vi "SLSC Add Status Section.vi"(5 "GUID Channel Interface":string="03D3BB89-1485-13A6-56005DE6430FF8B7", 6 "SLSC Channel Path":string="SLSCChannelPath", 7 "GUID (Default Section)":string="03D3BB89-1485-13A6-56005DE6430FF8B7", 8 "error in (no error)":errorcluster, 9 "Outgoing configuration":T3(array[cluster]), 10 "Section Name":string, 11 "Parent Ref in":T4 format="%.0x") -> (0 "error out":errorcluster, 3 "Parent Ref out":T4 format="%.0x")   [LabVIEW 2017, in "SLSC CD System Explorer.lvlib"]
uses:
  SLSC CD System Explorer.lvlib
  <vilib>/NI Veristand/Custom Device API/Custom Device Item Ref.ctl
  <vilib>/NI Veristand/Custom Device API/Custom Device Channel.ctl
  <vilib>/NI Veristand/Custom Device API/Custom Device Channel Type.ctl
  <vilib>/NI Veristand/Custom Device API/Set Item Property (String).vi
  <vilib>/NI VeriStand/Custom Device API/Custom Device API.lvlib
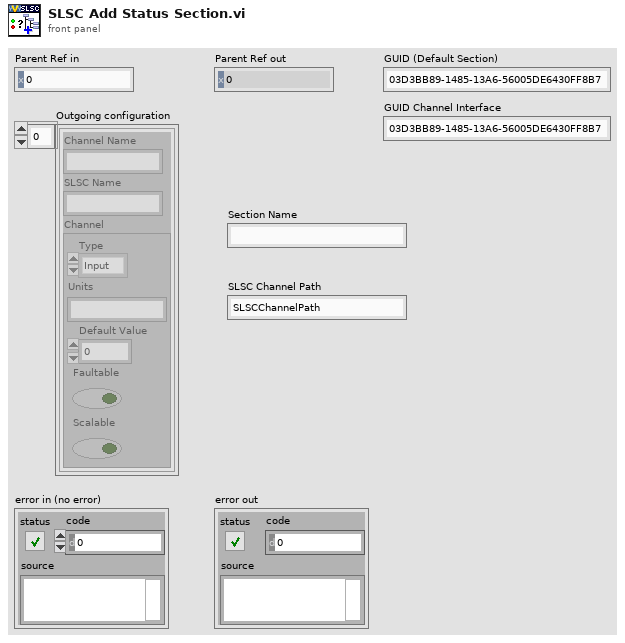
[diagram p1: front panel]
types:
  T1 = typedef "Custom Device API.lvlib/Custom Device Channel.ctl" = cluster{"Type":T2, "Units":string, "Default Value":dbl, "Faultable":bool, "Scalable":bool}
  T2 = typedef "Custom Device API.lvlib/Custom Device Channel Type.ctl" = enum16{"Input", "Output"}
  T3 = cluster{"Channel Name":string, "SLSC Name":string, "Channel":T1}[]
  T4 = typedef "Custom Device API.lvlib/Custom Device Item Ref.ctl" = u64
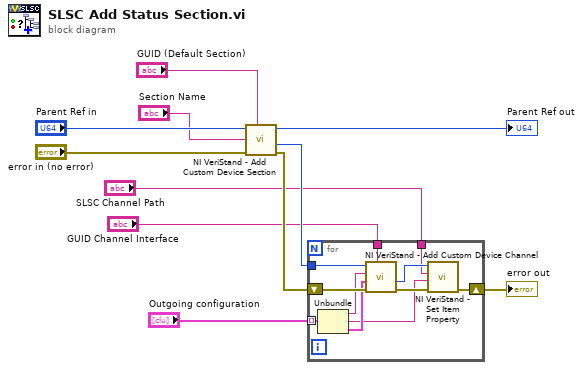
[diagram p0: block diagram]
diagram:
  n1 = call <vilib>:"NI VeriStand - Add Custom Device Section.vi"("GUID (Default Section)"="GUID (Default Section)", "error in (no error)"="error in (no error)", "Section Name"="Section Name", "Parent Ref in"="Parent Ref in") -> ("error out"=w5:errorcluster, "Section Ptr"=w6:T4, "Parent Ref out"=→"Parent Ref out":T4)  [unwired: 4 in, 1 out]
  n2 = for {
    tunnel: w6 -> [w19]
    shift-right: [w20] -> w7
    shift-left: w5 -> [w18]
    tunnel: "Outgoing configuration" -> [w17] mode=indexing
    tunnel: "GUID Channel Interface" -> [w13]
    tunnel: "SLSC Channel Path" -> [w12]
    n3 = Unbundle(w17) -> ("Channel Name"=w16:string, "SLSC Name"=w14:string, "Channel"=w15:T1)
    n4 = call <vilib>:"NI VeriStand - Add Custom Device Channel.vi"("GUID (Default Channel)"=w13, "error in (no error)"=w18, "Channel"=w15, "Channel Name"=w16, "Parent Ref in"=w19) -> ("error out"=w21:errorcluster, "Channel Ref"=w22:T4)  [unwired: 3 in, 2 out]
    n5 = call-poly <vilib>:"NI VeriStand - Set Item Property.vi"("error in (no error)"=w21, "Value"=w14, "Property Name"=w12, "Item Ref in"=w22) -> ("error out"=w20:errorcluster)  [unwired: 5 in, 2 out]
  }
  "error out" <- w7
